vi "qualification test.vi"(6 "XYZTheta":dbl[](array[numeric])) -> (1 "Gantry":dbl[](array[numeric])=[1219.240705557797, 722.8421823618999, 52.864847366341415, 0.003106741190800654] format="%#_8g", 2 "Sum":dbl[](array[numeric])=[1219.30639899585, 722.8896830877354, 52.864847366341415, 0.003106741190800654] format="%#_8g")   [LabVIEW 2016]
uses:
  Classes/Controller/Camera/Camera Folder/Machine Vision.ctl
  <vilib>/Utility/file.llb/Write Delimited Spreadsheet (DBL).vi
  Classes/Controller/I-O/I-O Folder/I-O.lvclass
  Classes/Controller/Motion/Motion Folder/Motion.lvclass
  Classes/Controller/Camera/Camera Folder/Camera.lvclass
  Classes/Controller/Controller Folder/Controller.lvclass
panel:
  out "Numeric":dbl
  in  "On/Off":bool=TRUE
  in  "Vacuum":bool
  out "Record Times":i32
  in  "Channel":i32=20
  in  "Filename":path=path "test.lvm"
  in  "Record":bool
  in  "Go 2":bool
  in  "Z Go":bool
  in  "Position":dbl
  in  "Machine Vision":T1=enum."tpcb_hole"
  in  "Go":bool
  in  "Joystick":bool
  in  "Stop":bool
  out "Image":T2(plugin-control)
  out "Camera":dbl[](array[numeric])=[0.23163148760795593, 0.18427667021751404] format="%#_8g"
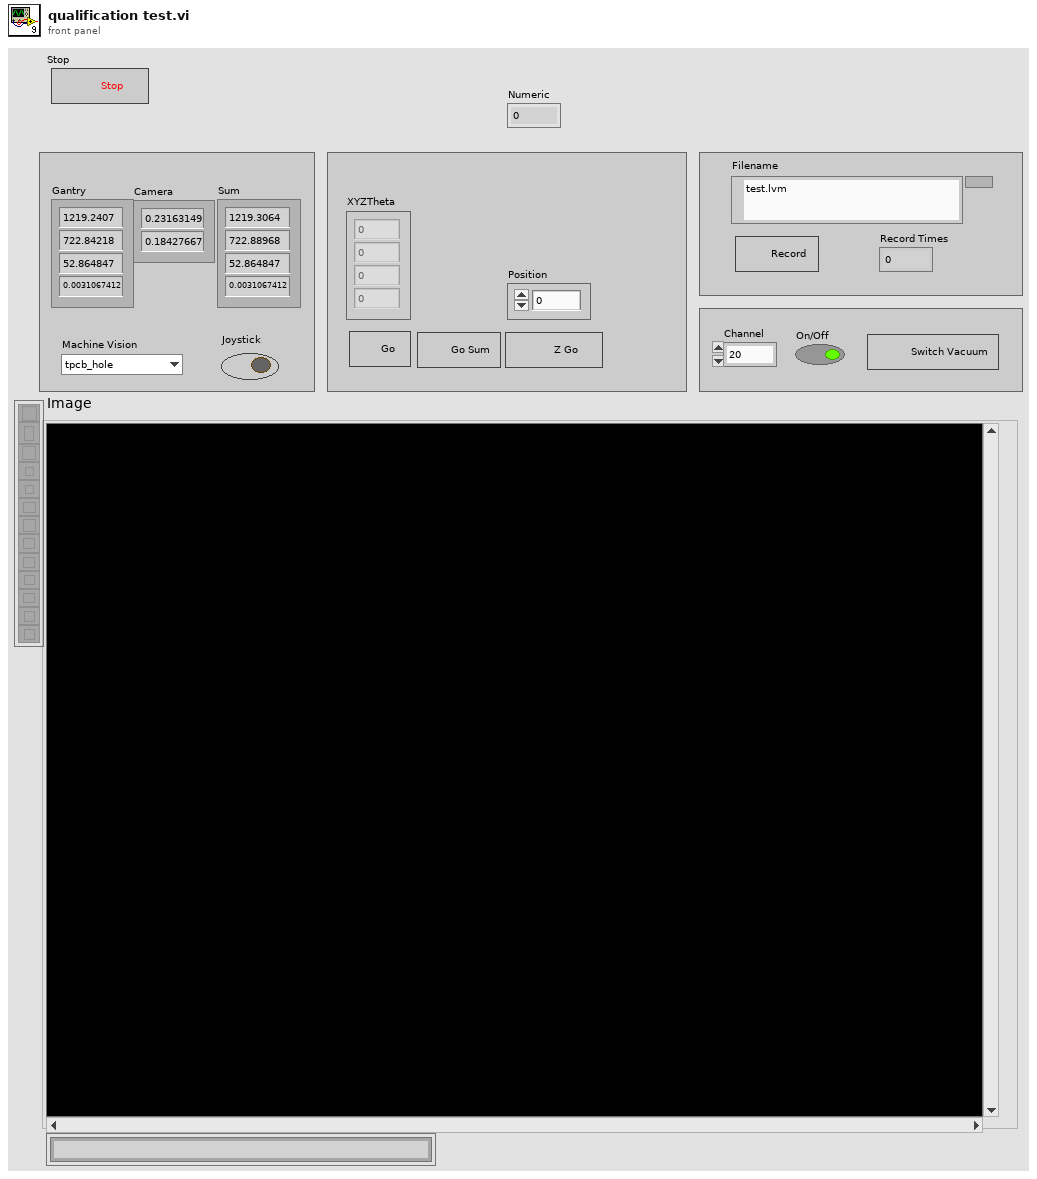
[diagram p1: front panel]
types:
  T1 = typedef "Camera.lvclass/Machine Vision.ctl" = enum16{"None", "Focus", "INTT HDI Mark", "INTT Sensor Cross", "INTT Chip Corner", "HPK Silicon", "Circle", "tpcb_hole"}
  T2 = typedef "IMAQ Image.ctl" = refnum<image>
  T3 = typedef "Controller.lvclass/Controllers.ctl" = cluster{"Copy of Motion.lvclass":refnum<class "Motion.lvclass">, "Copy of I-O.lvclass ":refnum<class "I-O.lvclass">, "Copy of Dispenser.lvclass":refnum<class "Dispenser.lvclass">}
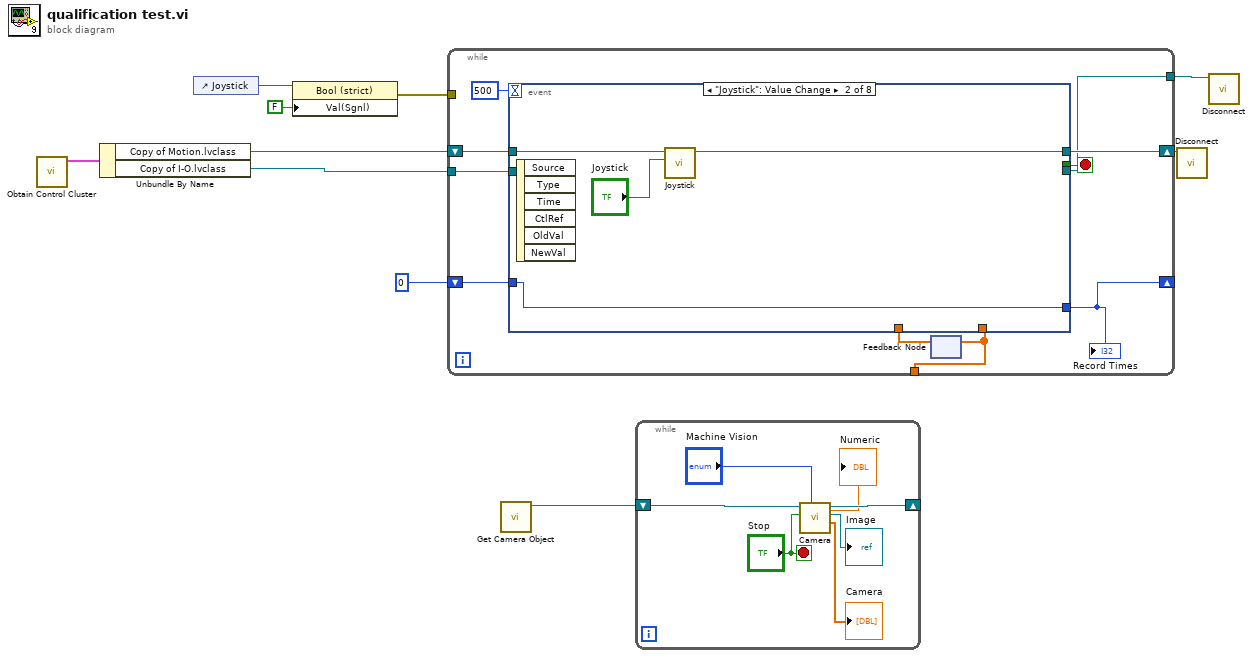
[diagram p0: block diagram]
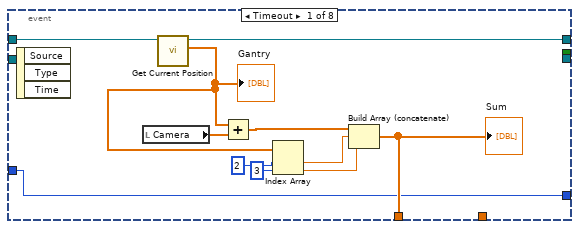
[diagram p2: hidden frame]
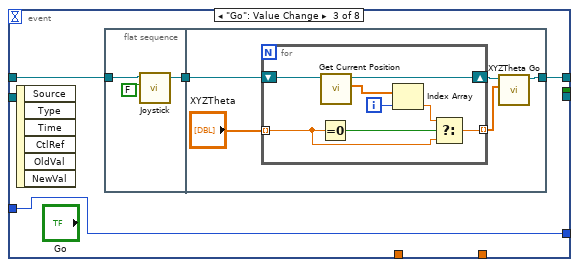
[diagram p3: hidden frame]
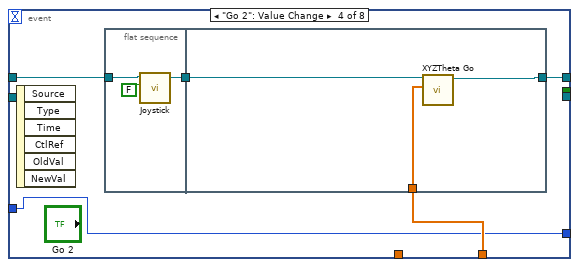
[diagram p4: hidden frame]
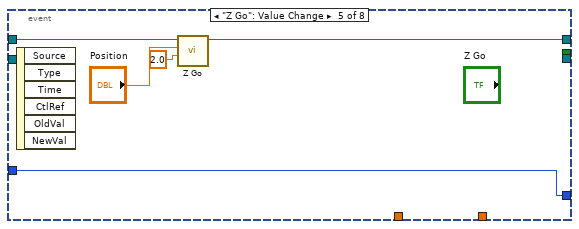
[diagram p5: hidden frame]
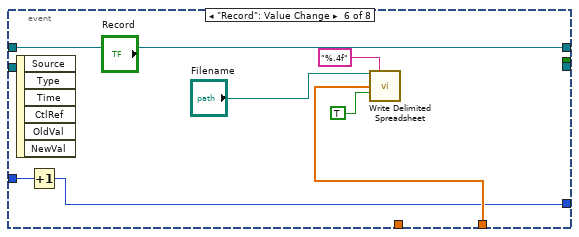
[diagram p6: hidden frame]
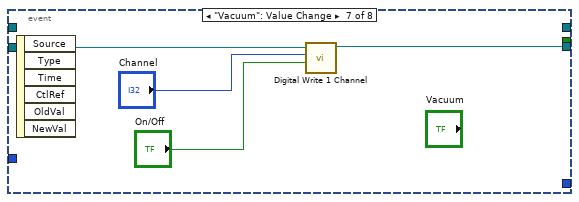
[diagram p7: hidden frame]
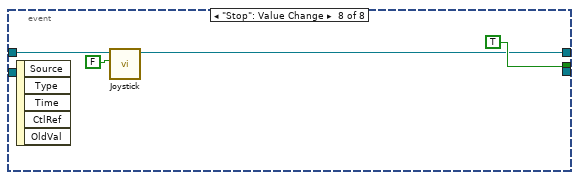
[diagram p8: hidden frame]
diagram:
  n1 = call "Obtain Control Cluster.vi"() -> ("Control Out"=w6:T3)  [unwired: 11 in]
  n2 = Unbundle By Name(w6) -> ("Copy of Motion.lvclass"=w5:refnum<class "Motion.lvclass">, "Copy of I-O.lvclass"=w1:refnum<class "I-O.lvclass">)
  n3 = control-ref of="Joystick"() -> (w9:refnum<vi>)
  n4 = property class="Bool (strict)"(reference=w9, "Val(Sgnl)"=FALSE ("Value (Signaling)")) -> (error out=w8:errorcluster)  [unwired: 1 in, 1 out]
  n5 = while {
    shift-right: [w18] -> w4
    shift-left: w5 -> [w15]
    tunnel: w8 -> [_]
    tunnel: [w17] -> _
    tunnel: w1 -> [w12]
    shift-right: [w13] -> _
    shift-left: 0 -> [w14]
    tunnel: [w11] -> w2
    stop <- w19 stop-if-true
    n6 = feedback #1() -> (w17:dbl[])  [unwired: 1 in]
    n7 = event shown="[1] \"Joystick\": Value Change" {
      selector: _ -> [_ _ _ _ _ _ _ _]
      dyn-events: _ -> [_ _ _ _ _ _ _ _]
      timeout: 500 -> [_ _ _ _ _ _ _ _]
      tunnel: [_ _ _ _ _ _ _ TRUE] -> w19
      tunnel: w15 -> [w30 w35 w39 w60 w71 w75 _ w85]
      tunnel: [w29 w33 w38 w59 w70 w75 _ w83] -> w18
      tunnel: [w25 _ _ _ _ _ _ _] -> w16
      tunnel: w17 -> [_ _ _ w57 _ w77 _ _]
      tunnel: w14 -> [w21 w32 w36 w56 w67 w73 _ _]
      tunnel: [w21 w32 w36 w56 w67 w72 _ _] -> w13
      tunnel: w12 -> [_ _ _ _ _ _ w82 _]
      tunnel: [_ _ _ _ _ _ w81 _] -> w11
      event Timeout {
        n8 = event-data() -> ()  [unwired: 1 in, 3 out]
        n9 = local read "Camera"() -> (w31:dbl[])
        n10 = call-dynamic "Get Current Position.vi"("Motion in"=w30) -> ("XYZTheta Out"=w27:dbl[], "Motion out"=w29:refnum<class "Motion.lvclass">)  [unwired: 8 in, 1 out]
        "Gantry" <- w27
        n11 = Add(x=w27, y=w31) -> (x+y=w28:dbl[])
        n12 = Index Array(array=w27, index #1=2 ("index"), index #2=3 ("index")) -> (element #1=w23:dbl, element #2=w22:dbl)
        n13 = Build Array (concatenate)(w28, w23, w22) -> (w25:dbl[])
        "Sum" <- w25
      }
      event "Joystick": Value Change {
        n14 = event-data() -> ()  [unwired: 1 in, 6 out]
        n15 = call-dynamic "Joystick.vi"("Joystick"="Joystick", "Motion in"=w35) -> ("Motion out"=w33:refnum<class "Motion.lvclass">)  [unwired: 8 in, 1 out]
      }
      event "Go": Value Change {
        n16 = event-data() -> ()  [unwired: 1 in, 6 out]
        n17 = flat-sequence {
          tunnel: w39 -> [w41]
          tunnel: [w40] -> w37
          tunnel: [w43] -> w38
          tunnel: w37 -> [w46]
          frame #0 {
            n18 = call-dynamic "Joystick.vi"("Joystick"=FALSE, "Motion in"=w41) -> ("Motion out"=w40:refnum<class "Motion.lvclass">)  [unwired: 8 in, 1 out]
          }
          frame #1 {
            n19 = for {
              tunnel: "XYZTheta" -> [w53] mode=indexing
              tunnel: [w51] -> w45 mode=indexing
              shift-right: [w49] -> w44
              shift-left: w46 -> [w50]
              i -> [w55]
              n20 = Equal To 0?(x=w53) -> (x = 0?=w54:bool)
              n21 = call-dynamic "Get Current Position.vi"("Motion in"=w50) -> ("XYZTheta Out"=w48:dbl[], "Motion out"=w49:refnum<class "Motion.lvclass">)  [unwired: 8 in, 1 out]
              n22 = Index Array(array=w48, index=w55) -> (element=w52:dbl)
              n23 = Select(t=w52, s=w54, f=w53) -> (s? t:f=w51:dbl)
            }
            n24 = call "XYZTheta Go.vi"("XYZTheta In"=w45, "Motion in"=w44) -> ("Motion out"=w43:refnum<class "Motion.lvclass">)  [unwired: 7 in, 2 out]
          }
        }
      }
      event "Go 2": Value Change {
        n25 = event-data() -> ()  [unwired: 1 in, 6 out]
        n26 = flat-sequence {
          tunnel: w60 -> [w62]
          tunnel: [w61] -> w58
          tunnel: [w66] -> w59
          tunnel: w58 -> [w65]
          tunnel: w57 -> [w64]
          frame #0 {
            n27 = call-dynamic "Joystick.vi"("Joystick"=FALSE, "Motion in"=w62) -> ("Motion out"=w61:refnum<class "Motion.lvclass">)  [unwired: 8 in, 1 out]
          }
          frame #1 {
            n28 = call "XYZTheta Go.vi"("XYZTheta In"=w64, "Motion in"=w65) -> ("Motion out"=w66:refnum<class "Motion.lvclass">)  [unwired: 7 in, 2 out]
          }
        }
      }
      event "Z Go": Value Change {
        n29 = event-data() -> ()  [unwired: 1 in, 6 out]
        n30 = call-dynamic "Z Go.vi"("Speed"=2.0, "Position"="Position", "Motion in"=w71) -> ("Motion out"=w70:refnum<class "Motion.lvclass">)  [unwired: 7 in, 1 out]
      }
      event "Record": Value Change {
        n31 = event-data() -> ()  [unwired: 1 in, 6 out]
        n32 = Increment(x=w73) -> (x+1=w72:i32)
        n33 = call-poly <vilib>:"Write Delimited Spreadsheet.vi"("file path (dialog if empty)"="Filename", "format (%.3f)"="%.4f", "1D data"=w77, "append to file? (new file:F)"=TRUE) -> ()  [unwired: 10 in, 2 out]
      }
      event "Vacuum": Value Change {
        n34 = event-data() -> ()  [unwired: 1 in, 6 out]
        n35 = call-dynamic "Digital Write 1 Channel.vi"("Value"="On/Off", "Channel"="Channel", "I-O.lvclass"=w82) -> ("I-O.lvclass 2"=w81:refnum<class "I-O.lvclass">)  [unwired: 7 in, 1 out]
      }
      event "Stop": Value Change {
        n36 = event-data() -> ()  [unwired: 1 in, 5 out]
        n37 = call-dynamic "Joystick.vi"("Joystick"=FALSE, "Motion in"=w85) -> ("Motion out"=w83:refnum<class "Motion.lvclass">)  [unwired: 8 in, 1 out]
      }
    }
    "Record Times" <- w13
    n38 = feedback-in #1(w16) -> ()
  }
  n39 = call "Get Camera Object.vi"() -> ("Camera out"=w7:refnum<class "Camera.lvclass">)  [unwired: 10 in, 1 out]
  n40 = while {
    shift-right: [w92] -> _
    shift-left: w7 -> [w93]
    stop <- "Stop" stop-if-true
    n41 = call "Camera.vi"("Machine Vision"="Machine Vision", "Stop"="Stop", "Camera in"=w93) -> ("Camera"=→"Camera":dbl[], "Image"=→"Image":T2, "Camera out"=w92:refnum<class "Camera.lvclass">, "Numeric"=→"Numeric":dbl)  [unwired: 4 in, 1 out]
  }
  n42 = call-dynamic "Disconnect.vi"("Motion in"=w4) -> ()  [unwired: 9 in, 1 out]
  n43 = call-dynamic "Disconnect.vi"("I-O in"=w2) -> ()  [unwired: 9 in, 1 out]
